vi "Read Slave ID.vi"(8 "error in (no error)":errorcluster, 11 "MB_Serial_Master in":refnum<class "MB_Master_Serial.lvclass">) -> (0 "error out":errorcluster, 2 "Slave ID":u8=1, 3 "MB_Serial_Master out":refnum<class "MB_Master_Serial.lvclass">)   [LabVIEW 2016, in "MB Master.lvlib" / "MB_Master_Serial.lvclass"]
uses:
  MB_Master_Serial.lvclass
  MB_ADU/MB_ADU.lvclass
  MB_ADU_Serial/MB_ADU_Serial.lvclass
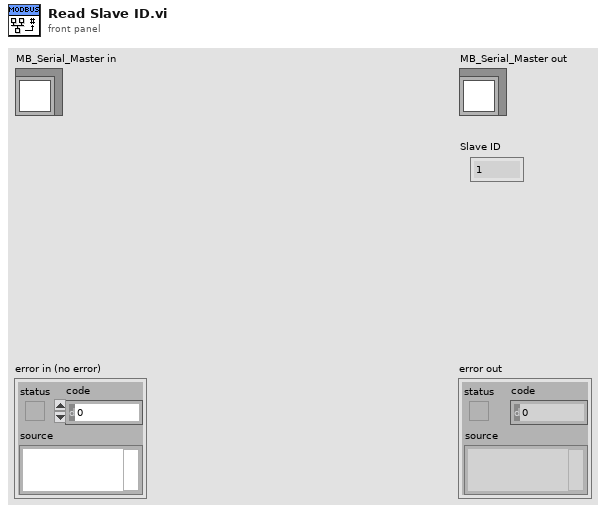
[diagram p1: front panel]
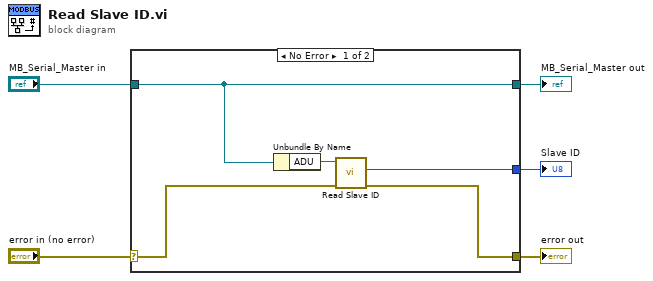
[diagram p0: block diagram]
diagram:
  n1 = case shown="No Error" "error in (no error)" {
    selector: "error in (no error)" -> [w9 w11]
    tunnel: [w8 w11] -> w4
    tunnel: [w6 w12] -> w2
    tunnel: "MB_Serial_Master in" -> [w6 w12]
    tunnel: [w7 _] -> w1
    frame No Error {
      n2 = Unbundle By Name(w6) -> ("ADU"=w10:refnum<class "MB_ADU_Serial.lvclass">)
      n3 = call "Read Slave ID.vi"("error in (no error)"=w9, "MB_ADU_Serial in"=w10) -> ("error out"=w8:errorcluster, "Slave Address"=w7:u8)  [unwired: 7 in, 1 out]
    }
    frame Error {
    }
  }
  "error out" <- w4
  "MB_Serial_Master out" <- w2
  "Slave ID" <- w1
